vi "MouseWheel Zoom Math.vi"(9 "Delta":i32, 10 "CursorPos":dbl, 11 "Range":T1) -> (3 "Range":T1)   [LabVIEW 2021, in "RocketPlot.lvlib"]
uses:
  RocketPlot.lvlib
  <vilib>/Utility/miscctls.llb/LVRangeTypeDef.ctl
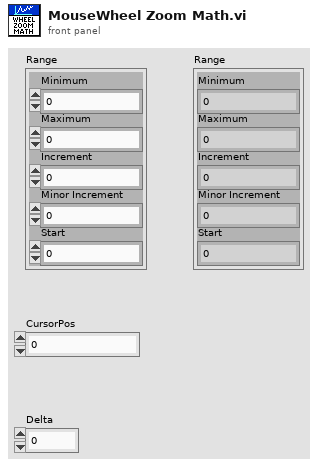
[diagram p1: front panel]
types:
  T1 = typedef "LVRangeTypeDef.ctl" = cluster{"Minimum":dbl, "Maximum":dbl, "Increment":dbl, "Minor Increment":dbl, "Start":dbl}
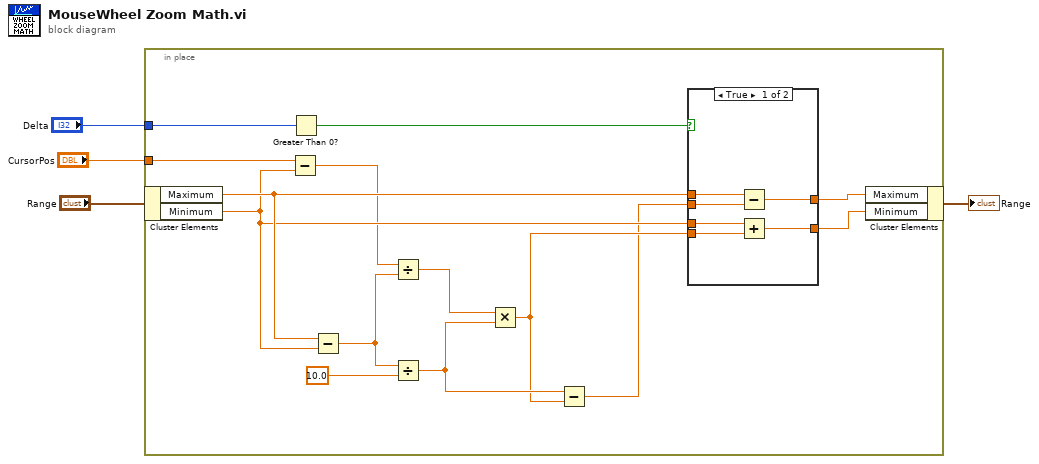
[diagram p0: block diagram]
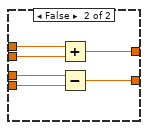
[diagram p2: hidden frame]
diagram:
  n1 = in-place {
    in-place-border: "CursorPos" -> [w10]
    in-place-border: "Delta" -> [w12]
    n2 = in-place-cluster #1("Range") -> ("Maximum"=w15:dbl, "Minimum"=w9:dbl)
    n3 = Subtract(x=w10, y=w9) -> (x-y=w8:dbl)
    n4 = Greater Than 0?(x=w12) -> (x > 0?=w11:bool)
    n5 = Subtract(x=w15, y=w9) -> (x-y=w18:dbl)
    n6 = Divide(x=w8, y=w18) -> (x/y=w17:dbl)
    n7 = Divide(x=w18, y=10.0) -> (x/y=w16:dbl)
    n8 = Multiply(x=w17, y=w16) -> (x*y=w7:dbl)
    n9 = Subtract(x=w16, y=w7) -> (x-y=w6:dbl)
    n10 = case shown="True" w11 {
      tunnel: w15 -> [w24 w30]
      tunnel: w6 -> [w23 w29]
      tunnel: w9 -> [w22 w28]
      tunnel: w7 -> [w21 w27]
      tunnel: [w20 w26] -> w14
      tunnel: [w19 w25] -> w13
      frame True {
        n11 = Subtract(x=w24, y=w23) -> (x-y=w20:dbl)
        n12 = Add(x=w22, y=w21) -> (x+y=w19:dbl)
      }
      frame False {
        n13 = Add(x=w30, y=w29) -> (x+y=w26:dbl)
        n14 = Subtract(x=w28, y=w27) -> (x-y=w25:dbl)
      }
    }
    n15 = in-place-cluster #1("Maximum"=w14, "Minimum"=w13) -> (→"Range":T1)
  }
